vi "DS18b20 Read.vi"(8 "error in (no error)":errorcluster) -> (0 "error out":errorcluster, 1 "found?":bool, 2 "ID":string, 3 "Temp":dbl)   [LabVIEW 2014, in "QwaveSys RPi Training Library.lvlib"]
uses:
  <vilib>/Q-Wave Systems/QwaveSys RPi Package 2.0/Addons/QwaveSys RPi Training Library.lvlib
  <vilib>/Q-Wave Systems/QwaveSys RPi Package 2.0/Addons/DS18b20/Ds18b20 ID.vi
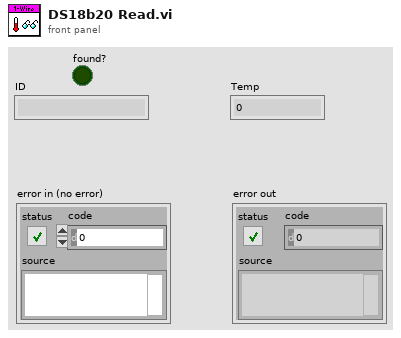
[diagram p1: front panel]
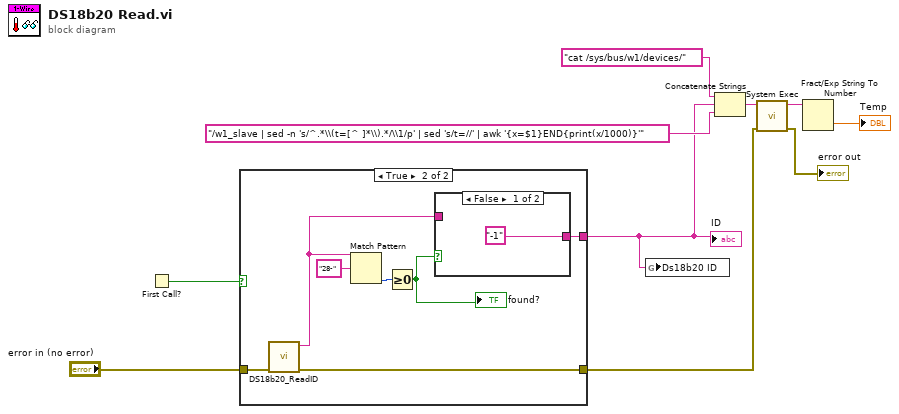
[diagram p0: block diagram]
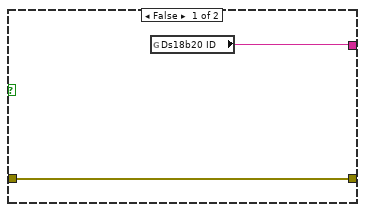
[diagram p2: hidden frame]
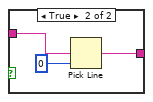
[diagram p3: hidden frame]
diagram:
  n1 = First Call?() -> (First Call?: T/F=w2:bool)
  n2 = case shown="True" w2 {
    tunnel: "error in (no error)" -> [w12 w15]
    tunnel: [w12 w14] -> w4
    tunnel: [w11 w13] -> w1
    frame False {
      n3 = global read "Ds18b20 ID.vi" "Ds18b20 ID"() -> (w11:string)
    }
    frame True {
      n4 = call <vilib>:"DS18b20_ReadID.vi"("error in (no error)"=w15) -> ("error out"=w14:errorcluster, "standard output"=w17:string)  [unwired: 9 in]
      n5 = Match Pattern(string=w17, regular expression="28-") -> (offset past match=w18:i32)  [unwired: 1 in, 3 out]
      n6 = Greater Or Equal To 0?(x=w18) -> (x >= 0?=w16:bool)
      "found?" <- w16
      n7 = case shown="False" w16 {
        tunnel: w17 -> [_ w22]
        tunnel: ["-1" ("output string") w21] -> w13
        frame False {
        }
        frame True {
          n8 = Pick Line(multi-line string=w22, line index=0) -> (output string=w21:string)  [unwired: 1 in]
        }
      }
    }
  }
  "ID" <- w1
  n9 = global write "Ds18b20 ID.vi" "Ds18b20 ID"(w1) -> ()
  n10 = Concatenate Strings("cat /sys/bus/w1/devices/" ("command line"), w1, "/w1_slave | sed -n 's/^.*\\(t=[^ ]*\\).*/\\1/p' | sed 's/t=//' | awk '{x=$1}END{print(x/1000)}'" ("command line")) -> (w10:string)
  n11 = call <vilib>:"System Exec.vi"("error in (no error)"=w4, "command line"=w10) -> ("error out"=→"error out":errorcluster, "standard output"=w7:string)  [unwired: 6 in, 2 out]
  n12 = Fract/Exp String To Number(string=w7) -> (number=→"Temp":dbl)  [unwired: 3 in, 1 out]
